vi "ComputeRasterCoordinatesAtAngle.vi"(7 "Antenna Angle":dbl, 8 "TestZT":cluster{"Z mm":dbl, "Horizontal T deg":dbl}={"Z mm"=0.0, "Horizontal T deg"=77.0}, 9 "Center Vector, y and x":dbl[](array[numeric])=[241.68344120684625, 300.8076172317183], 10 "Points per side":dbl=16.0, 11 "Nyquist, mm":dbl=28.0) -> ()   [LabVIEW 2017]
doc: "This version is aligned to the motion axes.\nIf the antenna is rotated slightly, ~ 1 - 3 degrees, this raster does not have that rotation."
panel:
  out "sin(x)":dbl
  out "cos(x)":dbl
  out "XY Graph for evaluation":cluster{dbl[], dbl[]}[](graph)
  out "Position Array":T1(array[cluster])
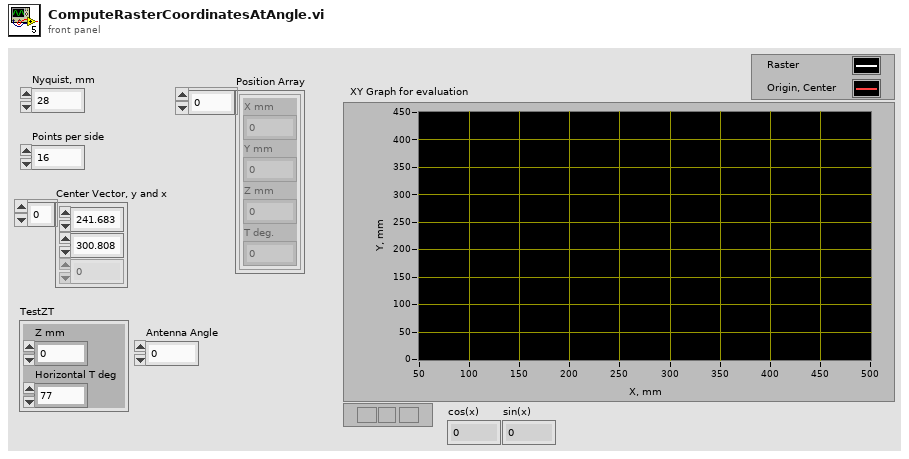
[diagram p1: front panel]
types:
  T1 = cluster{"X mm":dbl, "Y mm":dbl, "Z mm":dbl, "T deg.":dbl}[]
  T2 = cluster{"X mm":dbl, "Y mm":dbl, "Z mm":dbl, "T deg.":dbl}
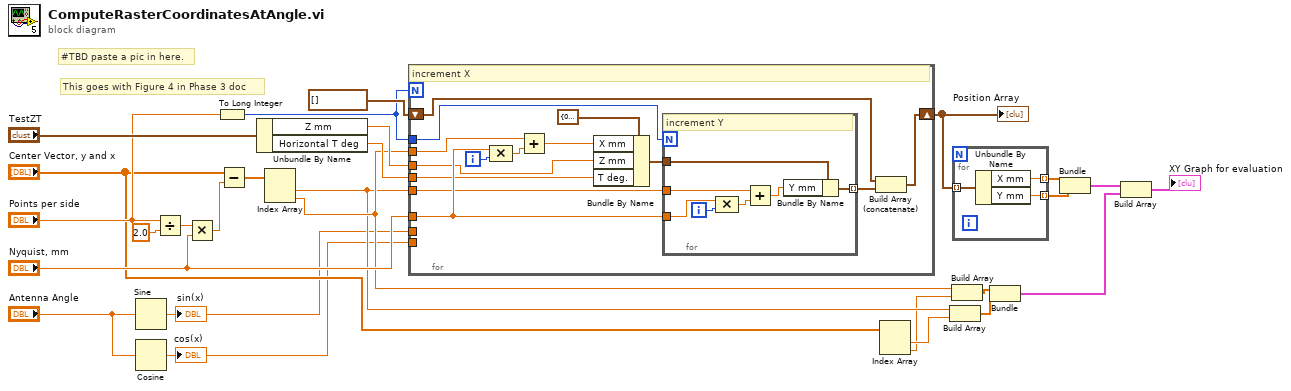
[diagram p0: block diagram]
diagram:
  # "#TBD paste a pic in here."
  # "This goes with Figure 4 in Phase 3 doc"
  n1 = Sine(x="Antenna Angle") -> (sin(x)=w2:dbl)
  "sin(x)" <- w2
  n2 = Cosine(x="Antenna Angle") -> (cos(x)=w1:dbl)
  "cos(x)" <- w1
  n3 = Divide(x="Points per side", y=2.0) -> (x/y=w22:dbl)
  n4 = Multiply(x=w22, y="Nyquist, mm") -> (x*y=w26:dbl)
  n5 = To Long Integer(number="Points per side") -> (32bit integer=w17:i32)
  n6 = Subtract(x="Center Vector, y and x", y=w26) -> (x-y=w21:dbl[])
  n7 = Unbundle By Name("TestZT") -> ("Z mm"=w23:dbl, "Horizontal T deg"=w20:dbl)
  n8 = Index Array(array=w21) -> (element #1=w11:dbl, element #2=w12:dbl)  [unwired: 2 in]
  n9 = for {
    N: w17 -> [_]
    tunnel: "Nyquist, mm" -> [w35]
    tunnel: w17 -> [w41]
    shift-right: [w40] -> w16
    shift-left: T1 [] -> [w39]
    tunnel: w23 -> [w32]
    tunnel: w20 -> [w31]
    tunnel: w11 -> [w34]
    tunnel: w12 -> [w30]
    tunnel: w2 -> [_]
    tunnel: w1 -> [_]
    i -> [w36]
    # "increment X"
    n10 = Compound Arithmetic op=MULTIPLY(w35, w36) -> (w37:dbl)
    n11 = Add(x=w30, y=w37) -> (x+y=w33:dbl)
    n12 = Bundle By Name(cluster=T2 {"X mm"=0.0, "Y mm"=0.0, "Z mm"=0.0, "T deg."=0.0} ("Position 15"), "X mm"=w33, "Z mm"=w32, "T deg."=w31) -> (w29:T2)
    n13 = for {
      N: w41 -> [_]
      tunnel: w34 -> [w48]
      tunnel: w35 -> [w46]
      tunnel: [w44] -> w38 mode=indexing
      tunnel: w29 -> [w42]
      i -> [w47]
      # "increment Y"
      n14 = Compound Arithmetic op=MULTIPLY(w46, w47) -> (w45:dbl)
      n15 = Add(x=w48, y=w45) -> (x+y=w43:dbl)
      n16 = Bundle By Name(cluster=w42, "Y mm"=w43) -> (w44:T2)
    }
    n17 = Build Array (concatenate)(w39, w38) -> (w40:T1)
  }
  "Position Array" <- w16
  n18 = Index Array(array="Center Vector, y and x") -> (element #1=w6:dbl, element #2=w5:dbl)  [unwired: 2 in]
  n19 = Build Array(w11, w6) -> (w9:dbl[])
  n20 = Build Array(w12, w5) -> (w10:dbl[])
  n21 = for {
    tunnel: w16 -> [w51] mode=indexing
    tunnel: [w50] -> w15 mode=indexing
    tunnel: [w49] -> w14 mode=indexing
    n22 = Unbundle By Name(w51) -> ("X mm"=w50:dbl, "Y mm"=w49:dbl)
  }
  n23 = Bundle(w10, w9) -> (w7:cluster{dbl[], dbl[]})  [unwired: 1 in]
  n24 = Bundle(w15, w14) -> (w13:cluster{dbl[], dbl[]})  [unwired: 1 in]
  n25 = Build Array(w13, w7) -> (→"XY Graph for evaluation":cluster{dbl[], dbl[]}[])
